vi "Format table.vi"(6 "error in (no error)":errorcluster, 8 "Table Control":string[][](table)=[["aaaa  ", "eeeee", "GGG", ""], ["bbb", "fffffffff", "", ""], ["ccccccc", "", "", ""], ["ddddddddd", "", "", ""], ["", "", "", "I"]], 9 "reference":refnum<vi>) -> (0 "error out":errorcluster)   [LabVIEW 2017]
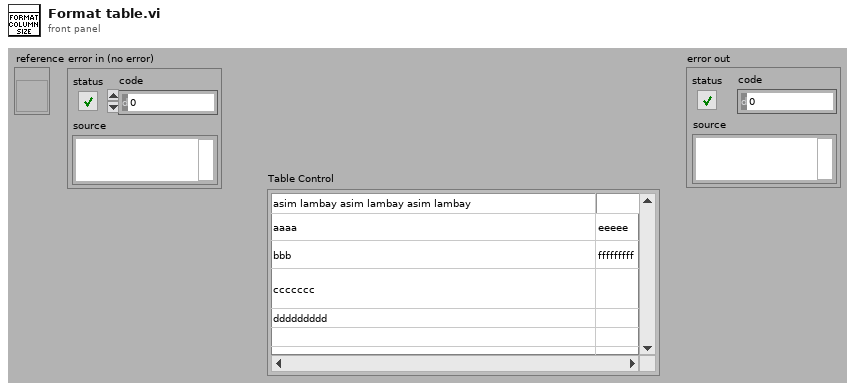
[diagram p1: front panel]
types:
  T1 = cluster{"Font Name:":string, "Size":i16, "Strikeout?":bool, "Italic?":bool, "Underline?":bool, "Outline?":bool, "Shadow?":bool, "Bold?":bool}
  T2 = enum16{"User-specified Font", "Application Font", "System Font", "Dialog Font"}
  T3 = typedef "LVFontTypeDef.ctl" = cluster{"Font Name":string, "Size":u16, "Bold":bool, "Italic":bool, "Underline":bool, "Strikeout":bool, "Color":u32}
  T4 = cluster{"left":i16, "top":i16, "right":i16, "bottom":i16}
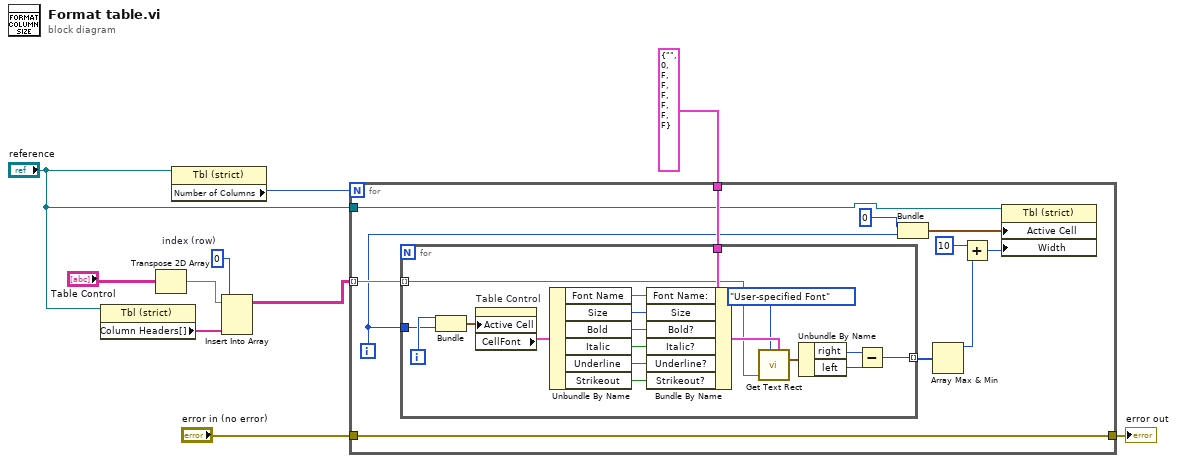
[diagram p0: block diagram]
diagram:
  w4 = 0  # index (row)
  n1 = property on="Property Node" class="Tbl (strict)"(reference="reference") -> ("Column Headers[]"=w5:string[])  [unwired: 1 in, 2 out]
  n2 = Transpose 2D Array(2D array="Table Control") -> (transposed array=w7:string[][])
  n3 = property on="Property Node" class="Tbl (strict)"(reference="reference") -> ("Number of Columns"=w10:u32)  [unwired: 1 in, 2 out]
  n4 = Insert Into Array(array=w7, index (row)=w4, new element=w5) -> (w6:string[][])  [unwired: 1 in]
  n5 = for {
    N: w10 -> [_]
    tunnel: w6 -> [w21] mode=indexing
    tunnel: T1 {"Font Name:"="", "Size"=0, "Strikeout?"=FALSE, "Italic?"=FALSE, "Underline?"=FALSE, "Outline?"=FALSE, "Shadow?"=FALSE, "Bold?"=FALSE} ("[user-specified font]") -> [w20]
    tunnel: "reference" -> [w12]
    tunnel: "error in (no error)" -> [w11]
    tunnel: [w11] -> w1
    i -> [w17]
    n6 = for {
      tunnel: w21 -> [w29] mode=indexing
      tunnel: w17 -> [w22]
      tunnel: w20 -> [w37]
      tunnel: [w24] -> w19 mode=indexing
      i -> [w23]
      n7 = Bundle(w23, w22) -> (w39:cluster{i32, i32})  [unwired: 1 in]
      n8 = property on="Table Control" class="Tbl (strict)"("Active Cell"=w39) -> ("CellFont"=w36:T3)  [unwired: 2 in, 2 out]
      n9 = Unbundle By Name(w36) -> ("Font Name"=w35:string, "Size"=w34:u16, "Bold"=w33:bool, "Italic"=w32:bool, "Underline"=w31:bool, "Strikeout"=w30:bool)
      n10 = Bundle By Name(cluster=w37, "Font Name:"=w35, "Size"=w34, "Bold?"=w33, "Italic?"=w32, "Underline?"=w31, "Strikeout?"=w30) -> (w38:T1)
      n11 = call <vilib>:"Get Text Rect.vi"("desired font(Application)"=T2."User-specified Font", "text"=w29, "[user-specified font]"=w38) -> ("rect"=w27:T4)  [unwired: 6 in]
      n12 = Unbundle By Name(w27) -> ("right"=w26:i16, "left"=w25:i16)
      n13 = Subtract(x=w26, y=w25) -> (x-y=w24:i16)
    }
    n14 = Bundle(0, w17) -> (w18:cluster{i32, i32})  [unwired: 1 in]
    n15 = Array Max & Min(array=w19) -> (max value=w13:i16)  [unwired: 3 out]
    n16 = Add(x=i16 10, y=w13) -> (x+y=w15:i16)
    n17 = property on="Property Node" class="Tbl (strict)"(reference=w12, "Active Cell"=w18, "Width"=w15) -> ()  [unwired: 1 in, 2 out]
  }
  "error out" <- w1
